vi "Destroy.vi"(11 "jettl Queue Actor in":refnum<class "jettl Queue Actor.lvclass">) -> (3 "jettl Queue Actor out":refnum<class "jettl Queue Actor.lvclass">)   [LabVIEW 2021, in "jettl Queue Actor.lvlib" / "jettl Queue Actor.lvclass"]
uses:
  jettl Queue Actor.lvclass
  C:/git/jettl/src/Actor/Actor/Actor.lvclass
  C:/git/jettl/src/Actor/Msgs/Setup/Setup/Setup.lvclass
  C:/git/jettl/src/Actor/Msgs/Teardown/Teardown/Teardown.lvclass
  C:/git/jettl/src/Actor/Queue Actor/Queue Actor.lvclass
  C:/git/jettl/src/Actor/Msgs/Event Create/Event Create/Event Create.lvclass
  C:/git/jettl/src/Actor/Msgs/Event Last Ack/Event Last Ack/Event Last Ack.lvclass
  C:/git/jettl/src/Actor/Msgs/Queue Create/Queue Create/Queue Create.lvclass
  C:/git/jettl/src/Actor/Msgs/Queue Last Ack/Queue Last Ack/Queue Last Ack.lvclass
  C:/git/jettl/src/jettl/jettl Queue Actor/jettl Queue Actor/jettl Queue Actor.lvclass
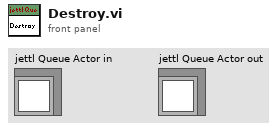
[diagram p1: front panel]
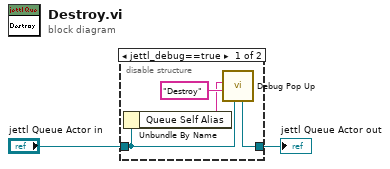
[diagram p0: block diagram]
diagram:
  n1 = disable-structure shown="jettl_debug==true" {
    disable-tunnel: "jettl Queue Actor in" -> [w4 _]
    disable-tunnel: [w5 _] -> w1
    frame condition #0 (active) {
      n2 = Unbundle By Name(w4) -> ("Queue Self Alias"=w3:string)
      n3 = call "Debug Pop Up.vi"("Input"=w4, "Method"="Destroy", "Alias"=w3) -> ("Output"=w5:refnum<class "jettl Queue Actor.lvclass">)  [unwired: 8 in]
    }
    frame condition #1 {
    }
  }
  "jettl Queue Actor out" <- w1
